vi "Servo ON_OFF.vi"(10 "Servo ON/OFF":bool) -> (2 "Command":string)   [LabVIEW 2017]
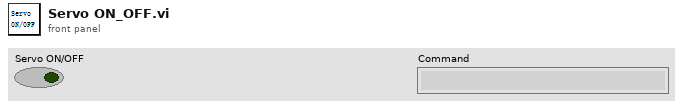
[diagram p1: front panel]
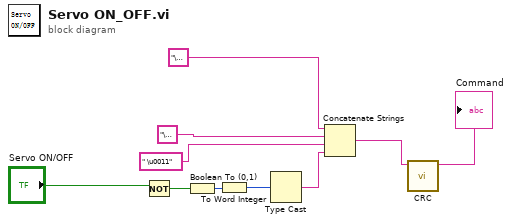
[diagram p0: block diagram]
diagram:
  n1 = Not(x="Servo ON/OFF") -> (.not. x?=w6:bool)
  n2 = Boolean To (0,1)(Boolean=w6) -> (0, 1=w5:i16)
  n3 = To Word Integer(number=w5) -> (16bit integer=w4:i16)
  n4 = Type Cast(x=w4) -> (*(type *) &x=w3:string)  [unwired: 1 in]
  n5 = Concatenate Strings("\u0001", "\u0006", " \u0011", w3) -> (w2:string)
  n6 = call "CRC.vi"("字符串"=w2) -> ("连接的字符串"=→"Command":string)  [unwired: 9 in, 1 out]
